vi "IQ Data to IO Node - S16.1 - N spc.vi"(0 "data in":T1[](array[typedef])=[{"I"=0.0, "Q"=0.0, "overflow"=FALSE}, {"I"=0.0, "Q"=0.0, "overflow"=FALSE}]) -> (4 "I out":fxp<+/-,16,1>[](array[numeric]), 6 "Q out":fxp<+/-,16,1>[](array[numeric]), 8 "overflow":bool[](array[boolean]))   [LabVIEW 2025, in "niUSRP Tx Core v1 FPGA.lvclass"]
doc: "For this Poly VI instance, 'data in' and 'data out' can support variable-sized arrays of 1 or 2 elements. The first element, data[0], is the oldest sample in the array.\n\nConverts a cluster of I/Q data into separate I and Q data in the fixed-point format, and indicates whether the I/Q data overflowed.\n\n<B>Input Parameters</B>\n\n<B>IQ data</B> specifies a bundle of real and imaginary data.\n\n<B>IQ data.I</B> specifies the bundled real data.\n\n<B>IQ data.Q</B> specifies the bundled imaginary data.\n\n<B>IQ data.overflow</B> specifies whether the I/Q data has overflowed.\n\n<B>Output Parameters</B>\n\n<B>fixed-point I data out</B> returns the real part of the data.\n\n<B>fixed-point Q data</B> returns the imaginary part of the data.\n\n<B>overflow</B> indicates whether the I/Q data has overflowed."
uses:
  niUSRP Tx Core v1 FPGA.lvclass
  <instrlib>/_niInstr/DSP/v1/Shared/Public/IQ Data.ctl
  <instrlib>/_niInstr/DSP/v1/Shared/niInstr DSP v1 Shared.lvlib
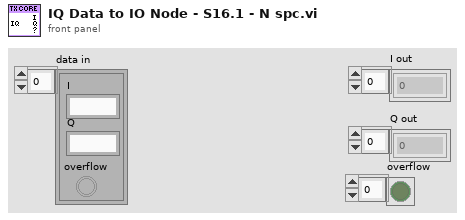
[diagram p1: front panel]
types:
  T1 = typedef "niInstr DSP v1 Shared.lvlib/IQ Data.ctl" = cluster{"I":fxp<+/-,18,1>, "Q":fxp<+/-,18,1>, "overflow":bool}
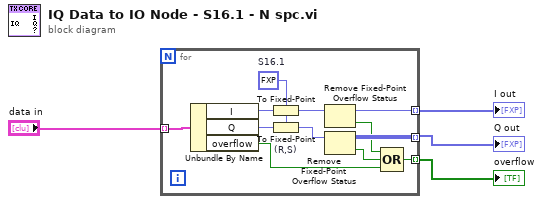
[diagram p0: block diagram]
diagram:
  n1 = for {
    tunnel: [w10] -> w4 mode=indexing
    tunnel: [w6] -> w2 mode=indexing
    tunnel: "data in" -> [w14] mode=indexing
    tunnel: [w8] -> w3 mode=indexing
    w13 = fxp<+/-,16,1> data[17B]  # S16.1
    n2 = Unbundle By Name(w14) -> ("I"=w16:fxp<+/-,18,1>, "Q"=w15:fxp<+/-,18,1>, "overflow"=w7:bool)
    n3 = To Fixed-Point(fixed-point type=w13, number=w16) -> (fixed-point=w11:fxp<+/-,16,1>)
    n4 = To Fixed-Point "(R,S)"(fixed-point type=w13, number=w15) -> (fixed-point=w9:fxp<+/-,16,1>)
    n5 = Remove Fixed-Point Overflow Status(3:w11) -> (0:w5:bool, 1:w10:fxp<+/-,16,1>)
    n6 = Remove Fixed-Point Overflow Status(3:w9) -> (0:w12:bool, 1:w6:fxp<+/-,16,1>)
    n7 = Compound Arithmetic op=OR(w5, w12, w7) -> (w8:bool)
  }
  "I out" <- w4
  "Q out" <- w2
  "overflow" <- w3
